vi "Create Test Queues.vi"(8 "error in (no error)":errorcluster, 11 "Generator in":refnum<class "Generator.lvclass">) -> (0 "error out":errorcluster, 3 "Generator out":refnum<class "Generator.lvclass">)   [LabVIEW 2019, in "Generator.lvclass"]
uses:
  Generator.lvclass
  typedefs/Waveforms--Cluster.ctl
  Generator.lvclass/Generator.ctl
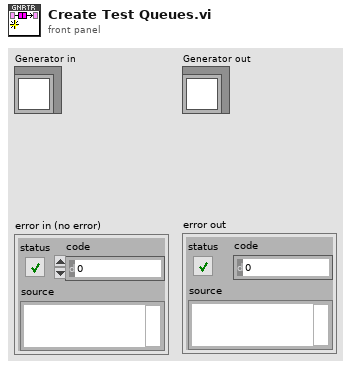
[diagram p1: front panel]
types:
  T1 = typedef "Generator.lvclass/Waveforms--Cluster.ctl" = cluster{"AO":waveform(dbl)[], "REF_X":waveform(dbl)[], "REF_Y":waveform(dbl)[]}
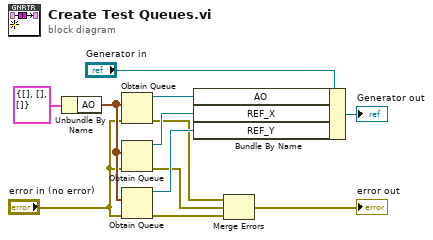
[diagram p0: block diagram]
diagram:
  n1 = Unbundle By Name(T1 {"AO"=[], "REF_X"=[], "REF_Y"=[]} ("Waveforms")) -> ("AO"=w7:waveform(dbl)[])
  n2 = Obtain Queue(element data type=w7, error in (no error)="error in (no error)") -> (queue out=w8:refnum<queue>, error out=w3:errorcluster)  [unwired: 3 in, 1 out]
  n3 = Obtain Queue(element data type=w7, error in (no error)="error in (no error)") -> (queue out=w11:refnum<queue>, error out=w1:errorcluster)  [unwired: 3 in, 1 out]
  n4 = Obtain Queue(element data type=w7, error in (no error)="error in (no error)") -> (queue out=w12:refnum<queue>, error out=w4:errorcluster)  [unwired: 3 in, 1 out]
  n5 = Bundle By Name(cluster="Generator in", "AO"=w8, "REF_X"=w11, "REF_Y"=w12) -> (→"Generator out":refnum<class "Generator.lvclass">)
  n6 = Merge Errors(w3, w1, w4) -> (→"error out":errorcluster)
